vi "StartTest.vi"(8 "error in (no error)":errorcluster, 11 "test_command":T1) -> (0 "error IO":errorcluster)   [LabVIEW 2018, in "Launcher Main Module.lvlib"]
uses:
  Launcher Main Module.lvlib
  Module_Controls/Test_Command.ctl
  TestStand_Control/TestStand_Control.lvlib
panel:
  out "TestCases":string[][](array[string])
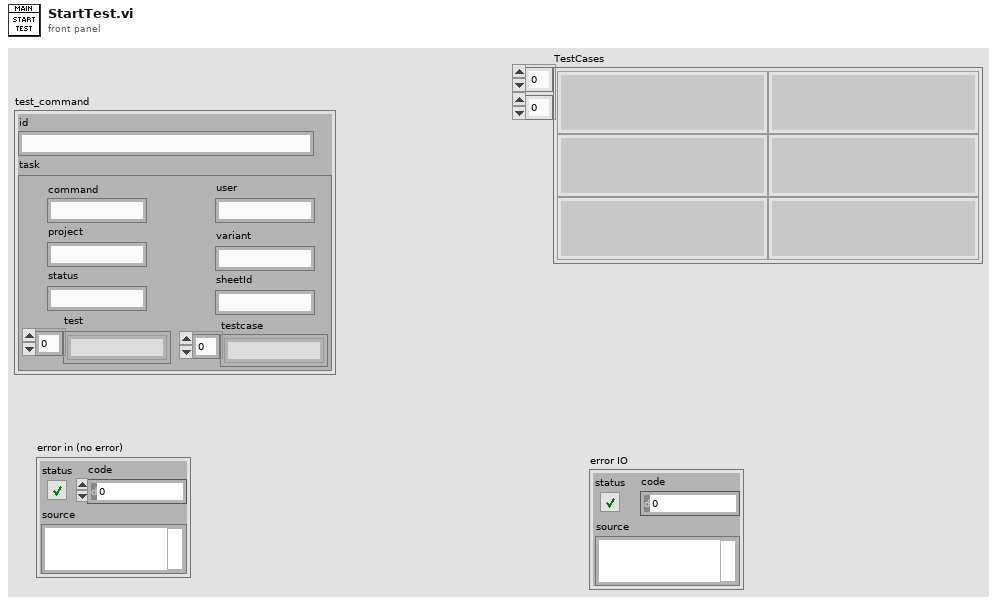
[diagram p1: front panel]
types:
  T1 = typedef "Launcher Main Module.lvlib/Test_Command.ctl" = cluster{"id":string, "task":cluster{"command":string, "project":string, "status":string, "sheetId":string, "test":string[], "user":string, "variant":string, "testcase":string[]}}
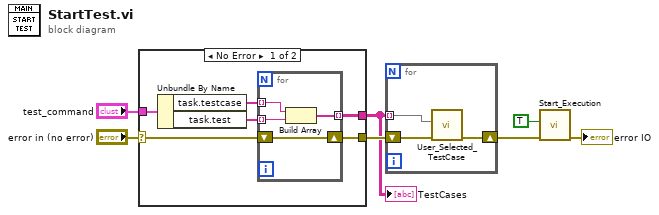
[diagram p0: block diagram]
diagram:
  n1 = case shown="No Error" "error in (no error)" {
    selector: "error in (no error)" -> [w12 w18]
    tunnel: [w10 w18] -> w5
    tunnel: "test_command" -> [w13 _]
    tunnel: [w9 _] -> w4
    frame No Error {
      n2 = Unbundle By Name(w13) -> ("task.testcase"=w11:string[], "task.test"=w8:string[])
      n3 = for {
        tunnel: w11 -> [w15] mode=indexing
        tunnel: [w16] -> w9 mode=indexing
        shift-right: [w17] -> w10
        shift-left: w12 -> [w17]
        tunnel: w8 -> [w14] mode=indexing
        n4 = Build Array(w15, w14) -> (w16:string[])
      }
    }
    frame Error {
    }
  }
  "TestCases" <- w4
  n5 = for {
    tunnel: w4 -> [w20] mode=indexing
    shift-right: [w19] -> w2
    shift-left: w5 -> [w21]
    n6 = call "User_Selected_TestCase.vi"("error in (no error)"=w21, "Test_Case_ID"=w20) -> ("error out"=w19:errorcluster)  [unwired: 9 in]
  }
  n7 = call "Start_Execution.vi"("error in (no error)"=w2, "Start"=TRUE) -> ("error out"=→"error IO":errorcluster)  [unwired: 9 in]
